vi "GOMDBTS2048 load Config.vi"(8 "error in (no error)":errorcluster, 10 "filename":string, 11 "handle":i32) -> (0 "error out":errorcluster, 3 "function return":i32)   [LabVIEW 2015, in "GOMDBTS2048.lvlib"]
doc: "GOBTS2048DLL int __stdcall GOMDBTS2048_loadConfig(int handle, char* filename);"
uses:
  GOMDBTS2048.lvlib
  runtime/GOMDBTS2048.dll
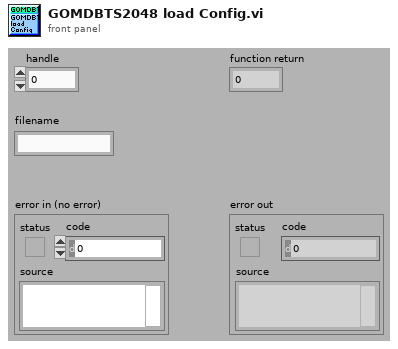
[diagram p1: front panel]
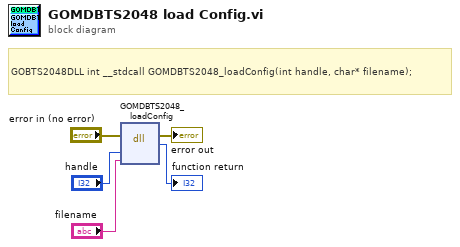
[diagram p0: block diagram]
diagram:
  # "GOBTS2048DLL int __stdcall GOMDBTS2048_loadConfig(int handle, char* filename);"
  n1 = dll-call lib="C:/Users/rkoch/Documents/GO_Library/runtime/GOMDBTS2048.*" fn="GOMDBTS2048_loadConfig"(error in="error in (no error)", "handle"="handle", "filename"="filename") -> (error out=→"error out":errorcluster, →"function return":i32)  [unwired: 4 in, 1 out]
